vi "Insight_RW_Fixed_Wavelength.vi"(7 "Parameter Type":enum16{"Value", "MAXimum", "MINimum", "DEFault"}(ring), 8 "error in (no error)":errorcluster, 9 "Mode (Read / Write)":enum8{"Write", "Read"}(ring), 10 "Wavelength (nm)":dbl=1520.0, 11 "telnet connection":T1) -> (0 "error out":errorcluster, 1 "response data":string, 2 "Wavelength (nm) ?":dbl, 3 "telnet  connection out":T1)   [LabVIEW 2015]
doc: "Insight Photonic Solutions\n\nThis reads or write the Fixed Wavelength to the laser, when in fixed wavelength mode.\n\nInputs:\nRead/Write : command or query the state of Fixed Wavelength Mode\nParameter Type - Tells the VI whether the command should use a Value or a keyword MAXimum, MINimum or DEFault to set the parameter value. (Default = Value).\nWavelength (nm): specify to within 1 picometer precision\n\nOutputs:\nResponse Data - Entire string response from the laser\nWavelength (nm)? - fixed wavelength value, in nm, parsed from the total strung response\n\nver 1.0 - original release\nver 3.3 - changed parser to handle responses from pre and post version 3.3 of Atlas\nver 3.4 - accepts key word values Max, Min or Default in addition to numeric values of the parameter"
uses:
  Telnet Session.ctl
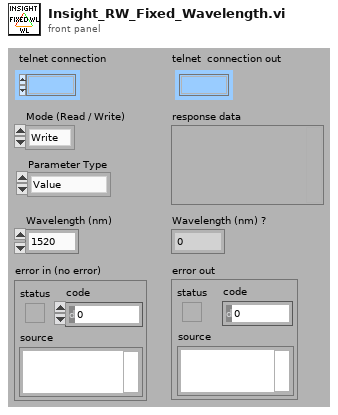
[diagram p1: front panel]
types:
  T1 = typedef "Telnet Session.ctl" = refnum<k1>
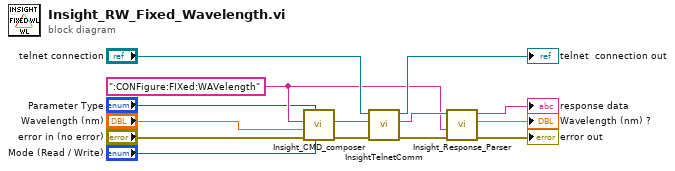
[diagram p0: block diagram]
diagram:
  w5 = ":CONFigure:FIXed:WAVelength" ("String")
  n1 = call "Insight_CMD_composer.vi"("Mode (Read / Write)"="Mode (Read / Write)", "Parameter Type"="Parameter Type", "error in (no error)"="error in (no error)", "Value"="Wavelength (nm)", "CMD"=w5) -> ("error out"=w7:errorcluster, "Command String"=w6:string)  [unwired: 5 in]
  n2 = call "InsightTelnetComm.vi"("error in"=w7, "write buffer (\"\")"=w6, "telnet connection"="telnet connection") -> ("error out"=w12:errorcluster, "response data"=w8:string, "telnet  connection out"=→"telnet  connection out":T1)  [unwired: 4 in]
  n3 = call "Insight_Response_Parser.vi"("error in (no error)"=w12, "Command String"=w5, "Laser Response In"=w8) -> ("error out"=→"error out":errorcluster, "Value"=→"Wavelength (nm) ?":dbl, "Laser Response Out"=→"response data":string)  [unwired: 6 in]
